vi "SetTBS2000.vi"(8 "error in (no error)":errorcluster, 10 "TBS2000Series":refnum<class "TBS2000Series.lvclass">, 11 "object in":refnum<class "Application.lvclass">) -> (0 "error out":errorcluster, 3 "object out":refnum<class "Application.lvclass">)   [LabVIEW 2023, in "Application.lvclass"]
uses:
  Application.lvclass
  Application.lvclass/Application.ctl
  TBS2000Series_class/TBS2000Series.lvclass
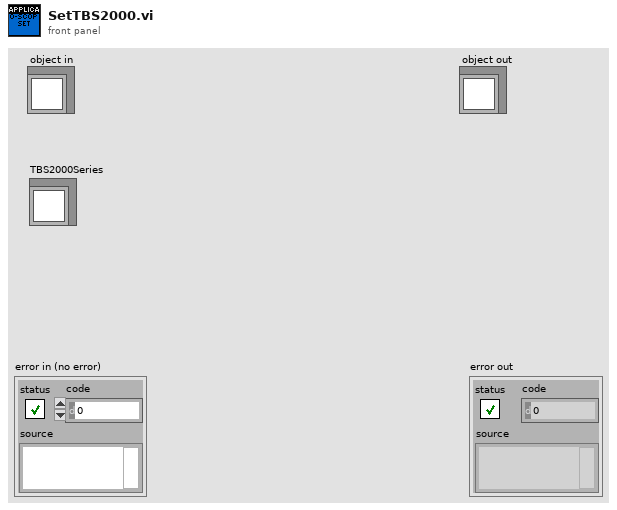
[diagram p1: front panel]
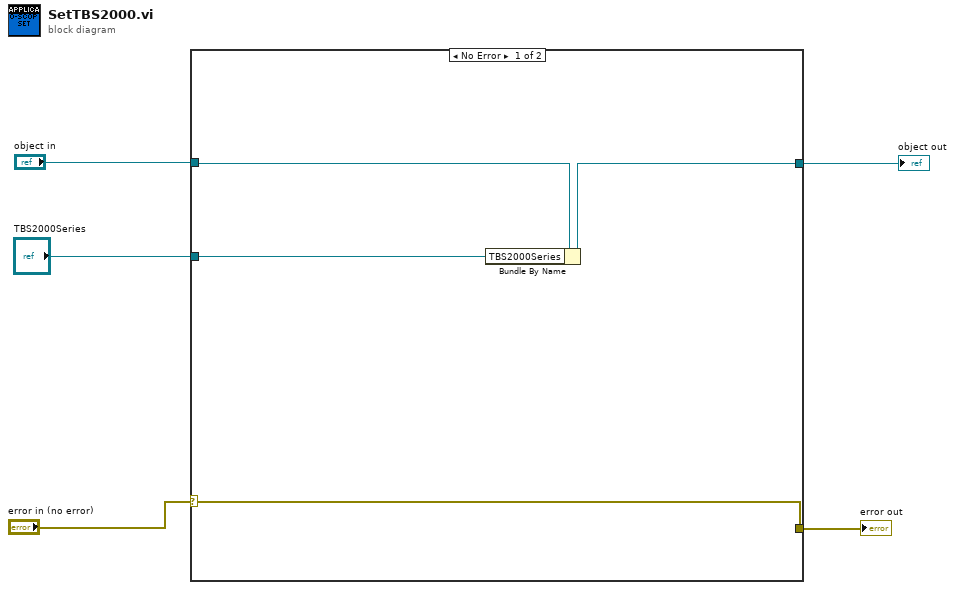
[diagram p0: block diagram]
diagram:
  n1 = case shown="No Error" "error in (no error)" {
    selector: "error in (no error)" -> [w8 w11]
    tunnel: [w8 w11] -> w4
    tunnel: [w6 w10] -> w3
    tunnel: "object in" -> [w7 w10]
    tunnel: "TBS2000Series" -> [w9 _]
    frame No Error {
      n2 = Bundle By Name(cluster=w7, "TBS2000Series"=w9) -> (w6:refnum<class "Application.lvclass">)
    }
    frame Error {
    }
  }
  "error out" <- w4
  "object out" <- w3
